vi "Encoder Loop.vi"(9 "Reset Position Value":i32, 10 "Reset Position":bool, 11 "Motor Module":T1={"Encoder Phase A"="Index1/Encoder Phase A", "Encoder Phase B"="Index1/Encoder Phase A", "Encoder Index"="Index1/Encoder Phase B"}) -> (0 "Index (Z) Position":i32, 1 "ticks/count":u32, 2 "counts (no reset)":i32, 3 "Encoder Position":i32)   [LabVIEW 2011]
uses:
  Controls/Encoder Module.ctl
  <vilib>/rvi/eio/common/nirviEmuTemplateMethod_errors.vi
  <vilib>/eio/EIONode/EIONode.xnode
panel:
  # "Use the Reset Position control to reset the quadrature count to the value in Reset Position Value."
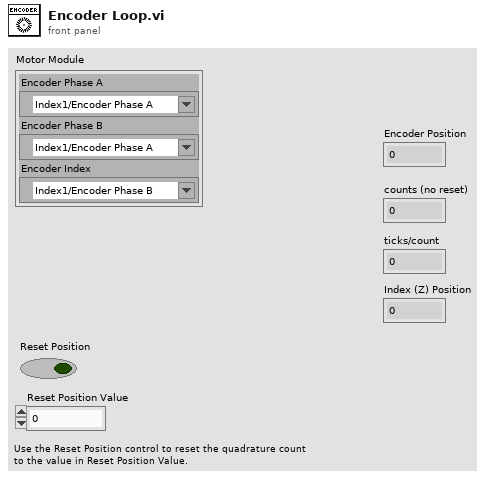
[diagram p1: front panel]
types:
  T1 = typedef "Encoder Module.ctl" = cluster{"Encoder Phase A":refnum<k21>, "Encoder Phase B":refnum<k21>, "Encoder Index":refnum<k21>}
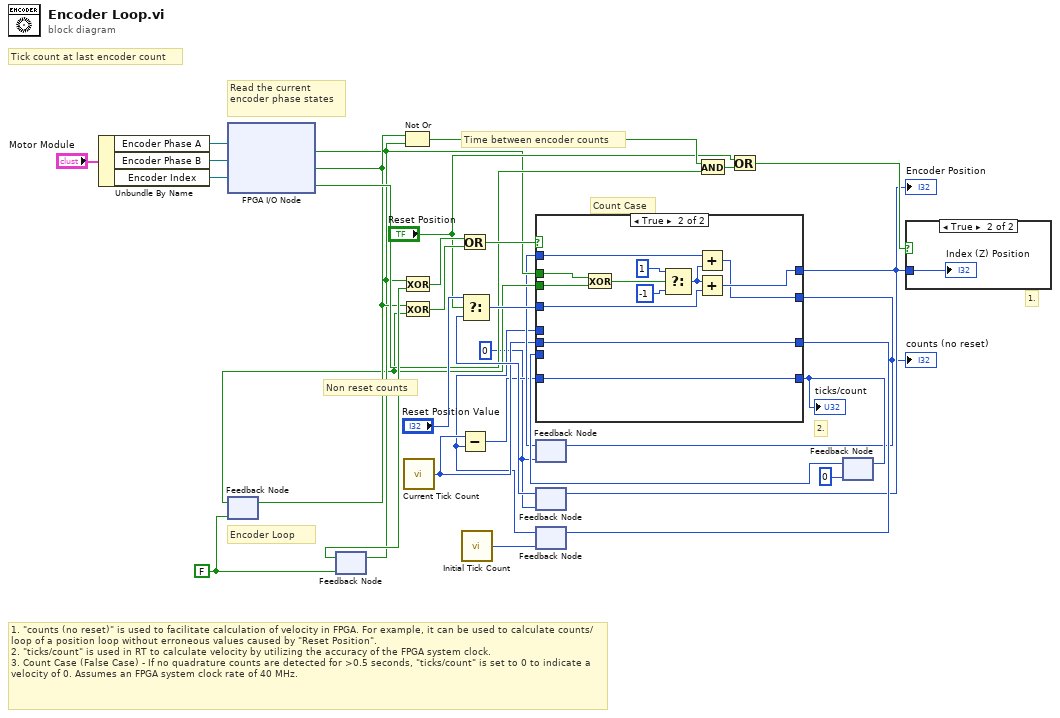
[diagram p0: block diagram]
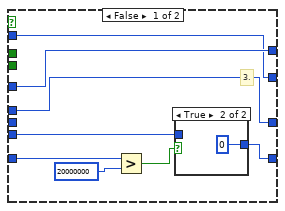
[diagram p3: hidden frame]
diagram:
  w1 = 0 ("Reset Position Value")
  w4 = FALSE ("Encoder Phase A")
  # "Count Case"
  # "Encoder Loop"
  # "2."
  # "1."
  # "Read the current\nencoder phase states"
  # "Non reset counts"
  # "Time between encoder counts"
  # "Tick count at last encoder count"
  # "1. \"counts (no reset)\" is used to facilitate calculation of velocity in FPGA. For example, it can be used to calculate counts/loop of a position loop without erroneous values caused by \"Reset Position\". \n2. \"ticks/count\" is used in RT to calculate velocity by utilizing the accuracy of the FPGA system clock.\n3. Count Case (False Case) - If no quadrature counts are detected for >0.5 seconds, \"ticks/count\" is set to 0 to indicate a velocity of 0. Assumes an FPGA system clock rate of 40 MHz."
  n1 = Unbundle By Name("Motor Module") -> ("Encoder Phase A"=w32:refnum<k21>, "Encoder Phase B"=w31:refnum<k21>, "Encoder Index"=w30:refnum<k21>)
  n2 = xnode "FPGA I/O Node"("FPGA I/O In"=w32, "FPGA I/O In"=w31, "FPGA I/O In"=w30) -> ("I/O Item"=w11:bool, "I/O Item"=w17:bool, "I/O Item"=w18:bool)  [unwired: 3 out]
  n3 = feedback #1(w4) -> (w10:bool)
  n4 = feedback-in #1(w17) -> ()
  n5 = feedback #2(w4) -> (w28:bool)
  n6 = feedback-in #2(w11) -> ()
  n7 = Not Or(1:w11, 2:w17) -> (0:w15:bool)
  n8 = Exclusive Or(1:w28, 2:w11) -> (0:w27:bool)
  n9 = Exclusive Or(1:w10, 2:w17) -> (0:w26:bool)
  n10 = call "Current Tick Count"() -> ("Tick Count(Ticks)"=w7:u32)
  n11 = Or(x=w27, y=w26) -> (x .or. y?=w24:bool)
  n12 = call "Initial Tick Count"() -> ("Tick Count(Ticks)"=w3:u32)
  n13 = feedback #3(w1) -> (w9:i32)
  n14 = feedback #4(w1) -> (w25:i32)
  n15 = Select(t="Reset Position Value", s="Reset Position", f=w25) -> (s? t:f=w23:i32)
  n16 = feedback #5(w3) -> (w6:u32)
  n17 = Subtract(x=w7, y=w6) -> (x-y=w5:u32)
  n18 = And(x=w15, y=w18) -> (x .and. y?=w16:bool)
  n19 = Or(x="Reset Position", y=w16) -> (x .or. y?=w14:bool)
  n20 = feedback #6(u32 0) -> (w19:u32)
  n21 = case shown="True" w24 {
    tunnel: [w40 w48] -> w13
    tunnel: w23 -> [w40 w54]
    tunnel: w7 -> [_ w44]
    tunnel: [w35 w44] -> w21
    tunnel: w6 -> [w35 _]
    tunnel: [w33 w43] -> w20
    tunnel: w19 -> [w34 _]
    tunnel: w11 -> [_ w50]
    tunnel: w10 -> [_ w49]
    tunnel: [w39 w46] -> w8
    tunnel: w9 -> [w39 w45]
    tunnel: w5 -> [w36 w43]
    frame False {
      # "3."
      n22 = Greater?(x=w36, y=20000000 ("x")) -> (0:w37:bool)
      n23 = case shown="True" w37 {
        tunnel: [w41 u32 0] -> w33
        tunnel: w34 -> [w41 _]
        frame False {
        }
        frame True {
        }
      }
    }
    frame True {
      n24 = Exclusive Or(1:w49, 2:w50) -> (0:w51:bool)
      n25 = Select(t=1 ("16 bit"), s=w51, f=-1 ("16 bit")) -> (s? t:f=w47:i32)
      n26 = Add(x=w45, y=w47) -> (x+y=w46:i32)
      n27 = Add(x=w47, y=w54) -> (x+y=w48:i32)
    }
  }
  "Encoder Position" <- w13
  "ticks/count" <- w20
  "counts (no reset)" <- w8
  n28 = feedback-in #3(w8) -> ()
  n29 = feedback-in #4(w13) -> ()
  n30 = feedback-in #5(w21) -> ()
  n31 = feedback-in #6(w20) -> ()
  n32 = case shown="True" w14 {
    tunnel: w13 -> [_ w55]
    frame False {
    }
    frame True {
      "Index (Z) Position" <- w55
    }
  }
